vi "SpreadsheetRead.vi"() -> (1 "Cluster":cluster{"X Array":dbl[], "Y Array":dbl[]})   [LabVIEW 2014]
uses:
  <vilib>/Utility/file.llb/Read From Spreadsheet File (DBL).vi
panel:
  out "XY Graph":cluster{"all rows":dbl[], "all rows":dbl[]}(graph)
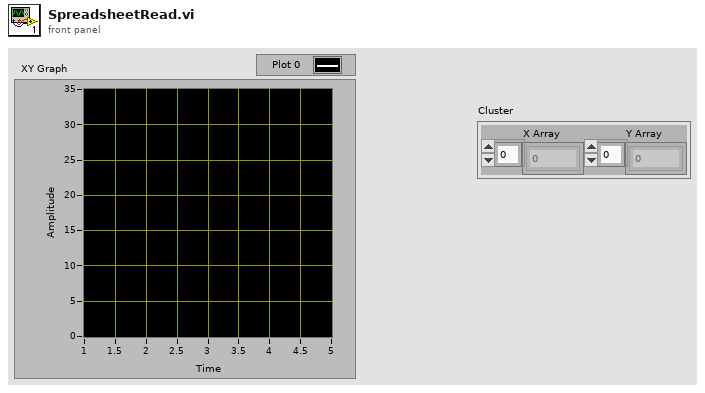
[diagram p1: front panel]
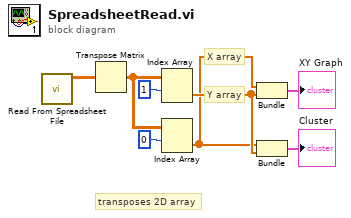
[diagram p0: block diagram]
diagram:
  # "Y array"
  # "X array"
  # "transposes 2D array"
  n1 = call-poly <vilib>:"Read From Spreadsheet File.vi"() -> ("all rows"=w7:dbl[][])  [unwired: 7 in, 4 out]
  n2 = Transpose Matrix(1:w7) -> (0:w6:dbl[][])
  n3 = Index Array(array=w6, index (row)=1) -> (element=w3:dbl[])  [unwired: 1 in]
  n4 = Index Array(array=w6, index (row)=0) -> (element=w2:dbl[])  [unwired: 1 in]
  n5 = Bundle("all rows"=w2, "all rows"=w3) -> (→"XY Graph":cluster{"all rows":dbl[], "all rows":dbl[]})  [unwired: 1 in]
  n6 = Bundle("all rows"=w2, "all rows"=w3) -> (→"Cluster":cluster{"all rows":dbl[], "all rows":dbl[]})  [unwired: 1 in]
